vi "Compare Dates.vi"(7 "Calibration Cycle (Days)":dbl, 9 "Last Cal Date":string, 11 "Current Date":string) -> (2 "Valid Cal?":bool)   [LabVIEW 2015]
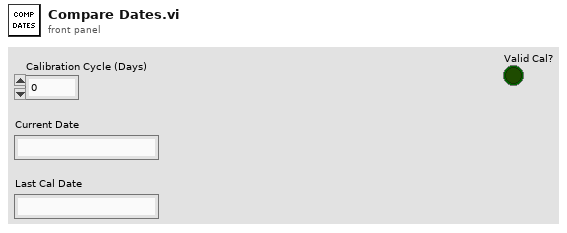
[diagram p1: front panel]
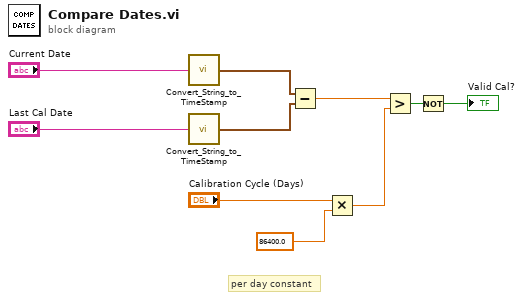
[diagram p0: block diagram]
diagram:
  # "per day constant"
  n1 = call "Convert_String_to_TimeStamp.vi"("date/time string"="Current Date") -> ("Resulting Time Stamp"=w8:timestamp)
  n2 = call "Convert_String_to_TimeStamp.vi"("date/time string"="Last Cal Date") -> ("Resulting Time Stamp"=w7:timestamp)
  n3 = Subtract(x=w8, y=w7) -> (x-y=w6:dbl)
  n4 = Multiply(x="Calibration Cycle (Days)", y=86400.0) -> (x*y=w2:dbl)
  n5 = Greater?(x=w6, y=w2) -> (0:w4:bool)
  n6 = Not(x=w4) -> (.not. x?=→"Valid Cal?":bool)
